vi "Clone Base Configuration.vi"(10 "Source Object":refnum<class "EMS Generic.lvclass">, 11 "Target Object in":refnum<class "EMS Generic.lvclass">) -> (3 "Target Object out":refnum<class "EMS Generic.lvclass">)   [LabVIEW 2018, in "EMS Generic Actor.lvlib" / "EMS Generic.lvclass"]
doc: "Takes all data stored in the source EMS Generic Object and places it in the target EMS Generic Object."
uses:
  EMS Generic.lvclass
  EMS Generic.lvclass/EMS Generic.ctl
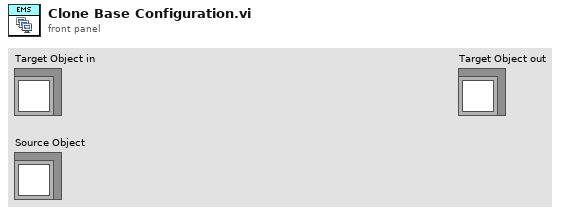
[diagram p1: front panel]
types:
  T1 = typedef "EMS Generic Actor.lvlib/EMS Generic.lvclass/Data Type DVRs.ctl" = cluster{"IED_Status":refnum<data-value>, "IED_Status_0":refnum<data-value>, "DER_Measurement":refnum<data-value>, "DER_Info":refnum<data-value>, "DER_Status":refnum<data-value>, "ES_Measurement":refnum<data-value>, "ES_Info":refnum<data-value>, "PV_Info":refnum<data-value>, "SmartRelay_Info":refnum<data-value>, "SmartRelay_Measurement":refnum<data-value>, "Meter_Info":refnum<data-value>, "Meter_Measurement":refnum<data-value>, "HVAC_Status":refnum<data-value>, "HVAC_Measurement":refnum<data-value>, "PriceData_RealTime":refnum<data-value>, "PriceData_Demand":refnum<data-value>, "PriceData_Energy":refnum<data-value>, "ForecastData_Long":refnum<data-value>, "ForecastData_Short":refnum<data-value>, "DER_Control":refnum<data-value>, "DER_SetPointF":refnum<data-value>, "DER_SetPointP":refnum<data-value>, "DER_SetPointQ":refnum<data-value>, "DER_SetPointPF":refnum<data-value>, "DER_SetPointV":refnum<data-value>, "PV_setCurtailment":refnum<data-value>, "PV_setRampRate":refnum<data-value>, "Relay_Control":refnum<data-value>, "Load_Control":refnum<data-value>, "HVAC_Control":refnum<data-value>, "Generator_Info":refnum<data-value>, "ForecastData_Long_Backup":refnum<data-value>, "PriceData_RealTime_Backup":refnum<data-value>}
  T2 = typedef "EMS Generic Actor.lvlib/EMS Generic.lvclass/Application Configuration.ctl" = cluster{"Log File Path":path, "Config File Path":path}
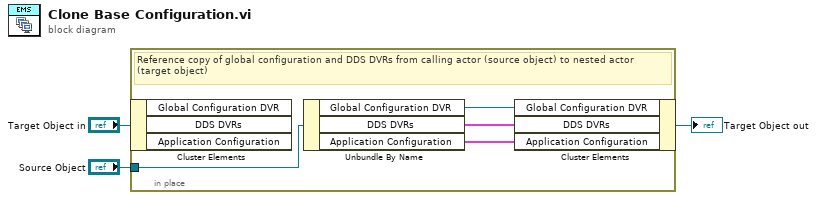
[diagram p0: block diagram]
diagram:
  n1 = in-place {
    in-place-border: "Source Object" -> [w7]
    # "Reference copy of global configuration and DDS DVRs from calling actor (source object) to nested actor (target object)"
    n2 = in-place-cluster #1("Target Object in") -> ()  [unwired: 3 out]
    n3 = Unbundle By Name(w7) -> ("Global Configuration DVR"=w6:refnum<data-value>, "DDS DVRs"=w5:T1, "Application Configuration"=w4:T2)
    n4 = in-place-cluster #1("Global Configuration DVR"=w6, "DDS DVRs"=w5, "Application Configuration"=w4) -> (→"Target Object out":refnum<class "EMS Generic.lvclass">)
  }
